vi "Digitizer Scale Ints.vi"(11 "Data Out":T1=[0, 0]) -> (3 "Array":T2)   [LabVIEW 2020]
doc: "Author: Scott Hannahs <sth@magnet.fsu.edu>\nCopyright 2018 Florida State University, All rights reserved."
uses:
  SCH Data Controls/SCH Secondary Int Data.ctl
  SCH Data Controls/SCH Raw Int Data Secondary.ctl
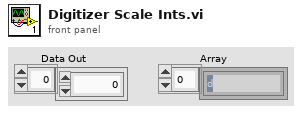
[diagram p1: front panel]
types:
  T1 = typedef "SCH Raw Int Data Secondary.ctl" = i16[]
  T2 = typedef "SCH Secondary Int Data.ctl" = fxp<+/-,19,5>[]
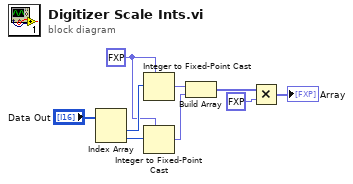
[diagram p0: block diagram]
diagram:
  w4 = fxp<+/-,16,1> 0.0 ("fixed-point type")
  n1 = Index Array(array="Data Out") -> (element #1=w6:i16, element #2=w5:i16)  [unwired: 2 in]
  n2 = Integer to Fixed-Point Cast(fixed-point type=w4, integer=w6) -> (fixed-point=w2:fxp<+/-,16,1>)
  n3 = Integer to Fixed-Point Cast(fixed-point type=w4, integer=w5) -> (fixed-point=w3:fxp<+/-,16,1>)
  n4 = Build Array(w2, w3) -> (w1:fxp<+/-,16,1>[])
  n5 = Multiply(x=w1, y=fxp<+,3,4> 10.0 ("fixed-point type")) -> (x*y=→"Array":fxp<+/-,19,5>[])
